vi "Joystick_PanelSim_Global.vi"(0 "menu":T4=enum."set left_rumble", 5 "JoystickDevice":T3, 7 "buttons":bool[](array[boolean]), 9 "Numeric Value":dbl format="%#.4f", 11 "error in (no error)":errorcluster, 12 "String Value":string, 13 "numbers":dbl[](array[numeric]) format="%#.4f") -> (10 "Joystick new":T1={"type"="Joystick", "device"="3", "name"="", "data"={"<init"=FALSE, ">buttons"=[], ">povs"=[], ">axes"=[], "<left_rumble"=0.0, "<right_rumble"=0.0, "<outputs"=0}}, 15 "error out":errorcluster)   [LabVIEW 2019]
doc: "This is used to set and get the last motor output values. This is needed for simulation, since we cannot read these values from the hardware.\n\nThis software is licensed. Open the labview\\readme\\WPI Robotics Library Open Source License.txt file for more information."
uses:
  Joystick Update Ops.ctl
  Joystick proto.ctl
  Joystick data proto.ctl
  <vilib>/Rock Robotics/WPI/Joystick/WPI_JoystickDeviceEnum.ctl
panel:
  out "All Values":T1[](array[typedef])
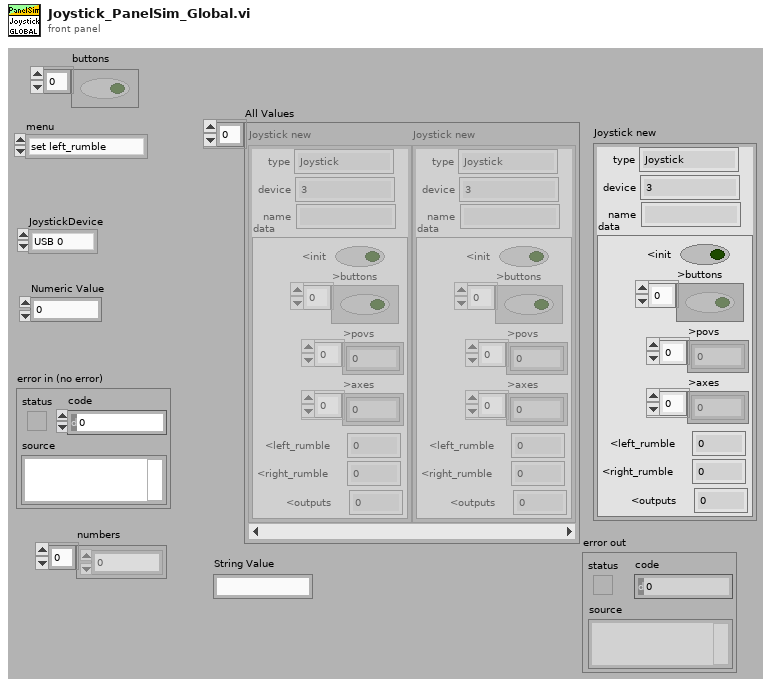
[diagram p1: front panel]
types:
  T1 = typedef "Joystick proto.ctl" = cluster{"type":string, "device":string, "name":string, "data":T2}
  T2 = typedef "Joystick data proto.ctl" = cluster{"<init":bool, ">buttons":bool[], ">povs":i32[], ">axes":i32[], "<left_rumble":dbl, "<right_rumble":dbl, "<outputs":i32}
  T3 = typedef "WPI_JoystickDeviceEnum.ctl" = enum16{"USB 0", "USB 1", "USB 2", "USB 3", "USB 4", "USB 5"}
  T4 = typedef "Joystick Update Ops.ctl" = enum16{"set init", "set buttons", "set povs", "set axes", "set left_rumble", "set right_rumble", "set outputs", "get", "delete", "JSON update", "set name", "transmit initial", "reset"}
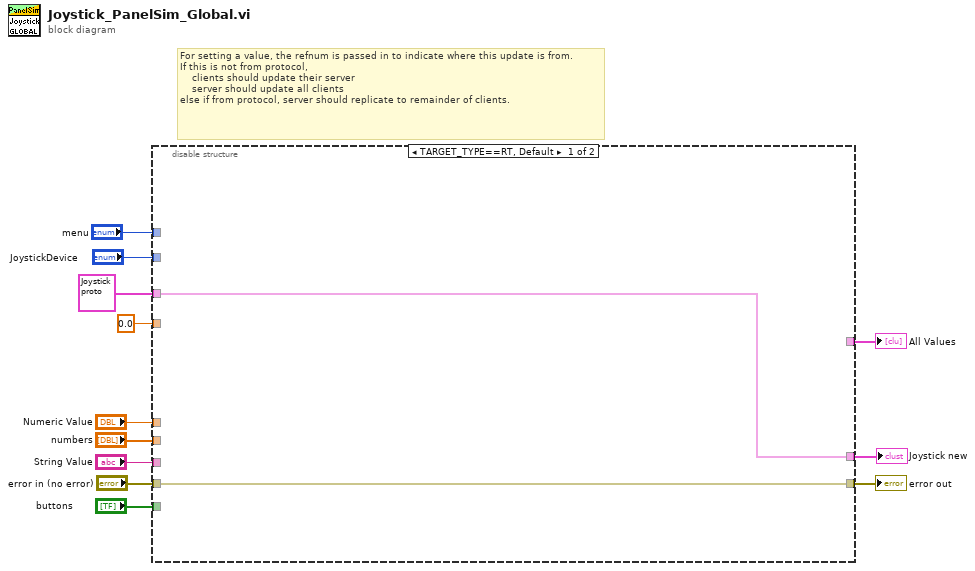
[diagram p0: block diagram]
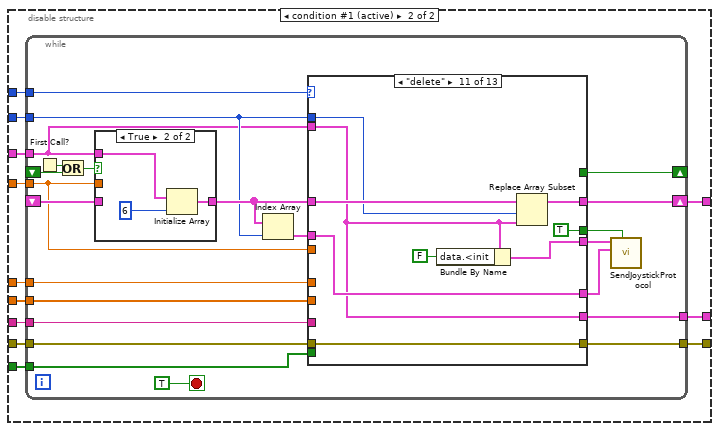
[diagram p2: hidden frame]
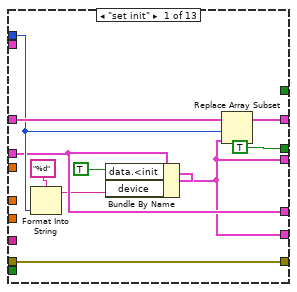
[diagram p3: hidden frame]
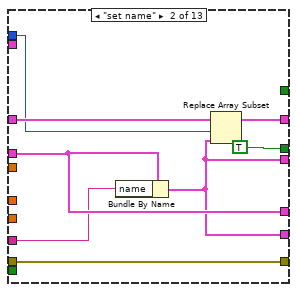
[diagram p4: hidden frame]
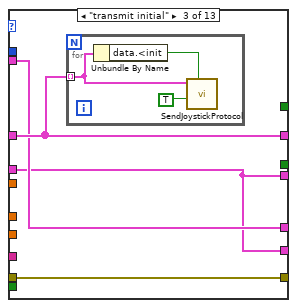
[diagram p5: hidden frame]
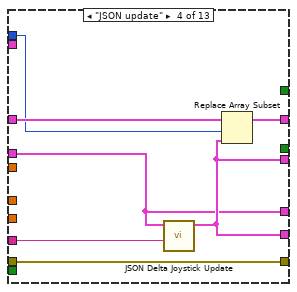
[diagram p6: hidden frame]
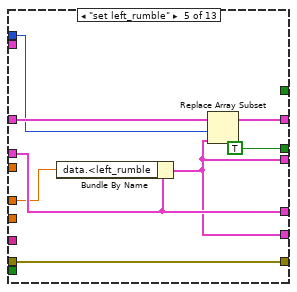
[diagram p7: hidden frame]
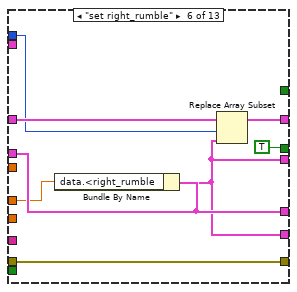
[diagram p8: hidden frame]
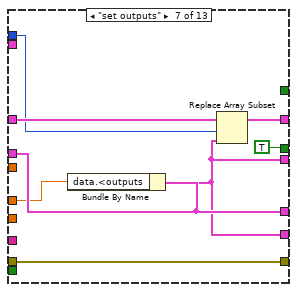
[diagram p9: hidden frame]
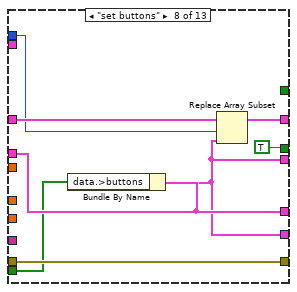
[diagram p10: hidden frame]
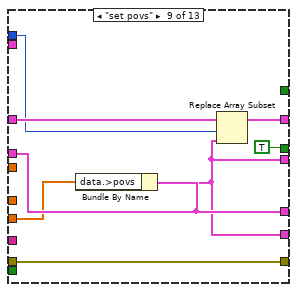
[diagram p11: hidden frame]
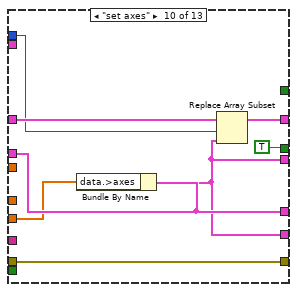
[diagram p12: hidden frame]
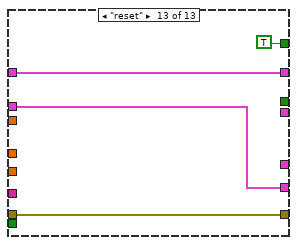
[diagram p14: hidden frame]
diagram:
  # "For setting a value, the refnum is passed in to indicate where this update is from.\nIf this is not from protocol,\n    clients should update their server\n    server should update all clients\nelse if from protocol, server should replicate to remainder of clients."
  n1 = disable-structure shown="TARGET_TYPE==RT, Default" {
    disable-tunnel: "menu" -> [_ w26]
    disable-tunnel: [w14 w25] -> w11
    disable-tunnel: "error in (no error)" -> [w14 w24]
    disable-tunnel: [_ w23] -> w9
    disable-tunnel: 0.0 ("Output") -> [_ w22]
    disable-tunnel: "JoystickDevice" -> [_ w21]
    disable-tunnel: [w13 w20] -> w6
    disable-tunnel: T1 {"type"="Joystick", "device"="3", "name"="", "data"={"<init"=FALSE, ">buttons"=[], ">povs"=[], ">axes"=[], "<left_rumble"=0.0, "<right_rumble"=0.0, "<outputs"=0}} ("Joystick new") -> [w13 w19]
    disable-tunnel: "String Value" -> [_ w18]
    disable-tunnel: "Numeric Value" -> [_ w17]
    disable-tunnel: "buttons" -> [_ w16]
    disable-tunnel: "numbers" -> [_ w15]
    frame condition #0 {
    }
    frame condition #1 (active) {
      n2 = while {
        tunnel: w24 -> [w46]
        shift-right: [w49] -> w23
        shift-left: _ -> [w42]
        tunnel: [w48] -> w20
        tunnel: w26 -> [w47]
        tunnel: [w45] -> w25
        tunnel: w21 -> [w40]
        tunnel: w22 -> [w41]
        tunnel: w19 -> [w39]
        tunnel: w18 -> [w38]
        tunnel: w17 -> [w37]
        tunnel: w16 -> [w36]
        tunnel: w15 -> [w31]
        shift-right: [w27] -> _
        shift-left: _ -> [w28]
        stop <- TRUE stop-if-true
        n3 = First Call?() -> (First Call?: T/F=w30:bool)
        n4 = Or(x=w30, y=w28) -> (x .or. y?=w29:bool)
        n5 = case shown="True" w29 {
          tunnel: [w146 w149] -> w43
          tunnel: w42 -> [w146 _]
          tunnel: w41 -> [_ _]
          tunnel: w39 -> [_ w148]
          frame False {
          }
          frame True {
            n6 = Initialize Array(w148, 6 ("dimension size")) -> (w149:T1[])
          }
        }
        n7 = Index Array(array=w43, index=w40) -> (element=w35:T1)
        n8 = case shown="\"delete\"" w47 {
          tunnel: [w59 w67 w70 w81 w89 w97 w105 w113 w121 w129 w137 w141 w145] -> w49
          tunnel: w43 -> [w57 w65 w70 w79 w87 w95 w103 w111 w119 w127 w138 w141 w145]
          tunnel: [w50 w61 w68 w77 w83 w91 w99 w107 w115 w123 w131 w139 w143] -> w48
          tunnel: [w58 w66 w71 w80 w88 w96 w104 w112 w120 w128 w136 w140 w144] -> w45
          tunnel: w46 -> [w58 w66 w71 w80 w88 w96 w104 w112 w120 w128 w136 w140 w144]
          tunnel: w40 -> [w54 w63 _ w78 w85 w93 w101 w109 w117 w125 w133 _ _]
          tunnel: w41 -> [_ _ _ _ _ _ _ _ _ _ _ _ _]
          tunnel: [w50 w61 w68 w77 w83 w91 w99 w107 w115 w123 w132 _ _] -> w32
          tunnel: [w53 w62 w69 w76 w84 w92 w100 w108 w116 w124 w134 _ _] -> w33
          tunnel: [TRUE TRUE _ _ TRUE TRUE TRUE TRUE TRUE TRUE TRUE _ _] -> w34
          tunnel: w35 -> [w53 w62 w68 w76 w84 w92 w100 w108 w116 w124 w134 w139 w143]
          tunnel: w39 -> [_ _ w69 _ _ _ _ _ _ _ w131 _ _]
          tunnel: w38 -> [_ w60 _ w75 _ _ _ _ _ _ _ _ _]
          tunnel: w37 -> [_ _ _ _ w82 w90 w98 _ _ _ _ _ _]
          tunnel: w36 -> [_ _ _ _ _ _ _ w106 _ _ _ _ _]
          tunnel: w31 -> [_ _ _ _ _ _ _ _ w114 w122 _ _ _]
          tunnel: [_ _ _ _ _ _ _ _ _ _ _ _ TRUE] -> w27
          frame "set init" {
            n9 = Format Into String(format string="%d", w54) -> (resulting string=w51:string)  [unwired: 2 in, 1 out]
            n10 = Bundle By Name(cluster=w53, "data.<init"=TRUE, "device"=w51) -> (w50:T1)
            n11 = Replace Array Subset(array=w57, new element=w50, index=w54) -> (w59:T1[])
          }
          frame "set name" {
            n12 = Bundle By Name(cluster=w62, "name"=w60) -> (w61:T1)
            n13 = Replace Array Subset(array=w65, new element=w61, index=w63) -> (w67:T1[])
          }
          frame "transmit initial" {
            n14 = for {
              tunnel: w70 -> [w73] mode=indexing
              n15 = Unbundle By Name(w73) -> ("data.<init"=w74:bool)
              n16 = call "SendJoystickProtocol.vi"("Send"=w74, "Initialize"=TRUE, "Joystick new"=w73) -> ()  [unwired: 9 in]
            }
          }
          frame "JSON update" {
            n17 = call "JSON Delta Joystick Update.vi"("Delta JSON"=w75, "input"=w76) -> ("output"=w77:T1)  [unwired: 8 in, 1 out]
            n18 = Replace Array Subset(array=w79, new element=w77, index=w78) -> (w81:T1[])
          }
          frame "set left_rumble" {
            n19 = Bundle By Name(cluster=w84, "data.<left_rumble"=w82) -> (w83:T1)
            n20 = Replace Array Subset(array=w87, new element=w83, index=w85) -> (w89:T1[])
          }
          frame "set right_rumble" {
            n21 = Bundle By Name(cluster=w92, "data.<right_rumble"=w90) -> (w91:T1)
            n22 = Replace Array Subset(array=w95, new element=w91, index=w93) -> (w97:T1[])
          }
          frame "set outputs" {
            n23 = Bundle By Name(cluster=w100, "data.<outputs"=w98) -> (w99:T1)
            n24 = Replace Array Subset(array=w103, new element=w99, index=w101) -> (w105:T1[])
          }
          frame "set buttons" {
            n25 = Bundle By Name(cluster=w108, "data.>buttons"=w106) -> (w107:T1)
            n26 = Replace Array Subset(array=w111, new element=w107, index=w109) -> (w113:T1[])
          }
          frame "set povs" {
            n27 = Bundle By Name(cluster=w116, "data.>povs"=w114) -> (w115:T1)
            n28 = Replace Array Subset(array=w119, new element=w115, index=w117) -> (w121:T1[])
          }
          frame "set axes" {
            n29 = Bundle By Name(cluster=w124, "data.>axes"=w122) -> (w123:T1)
            n30 = Replace Array Subset(array=w127, new element=w123, index=w125) -> (w129:T1[])
          }
          frame "delete" {
            n31 = Bundle By Name(cluster=w131, "data.<init"=FALSE) -> (w132:T1)
            n32 = Replace Array Subset(array=w138, new element=w131, index=w133) -> (w137:T1[])
          }
          frame "get" {
          }
          frame "reset" {
          }
        }
        n33 = call "SendJoystickProtocol.vi"("Send"=w34, "Joystick old"=w33, "Joystick new"=w32) -> ()  [unwired: 9 in]
      }
    }
  }
  "error out" <- w11
  "All Values" <- w9
  "Joystick new" <- w6
